vi "IL Turbo Speed.vi"(4 "Add to (Deny)":T1, 5 "Ignore (F)":bool, 6 "Range (>80%)":cluster{"Upper Limit":dbl, "Lower Limit":dbl}={"Upper Limit"=inf, "Lower Limit"=80.0}, 7 "Stop Self on IL? (T)":bool=TRUE, 8 "error in (no error)":errorcluster, 10 "IL Actions":refnum<class "IL Action.lvclass">[](array[class]), 11 "Interlock Chain in":refnum<class "Interlock Chain.lvclass">) -> (0 "error out":errorcluster, 2 "IL Turbo Valve":refnum<class "Interlock.lvclass">, 3 "Interlock Chain out":refnum<class "Interlock Chain.lvclass">)   [LabVIEW 2015, in "cRIO-Carbondioxide.lvlib" / "cRIO-CO2.lvlib" / "cRIO-CO2.lvclass"]
uses:
  cRIO-CO2.lvclass
  Interlocks/Interlock Chain/Interlock Chain.lvclass
  Interlocks/Controls/Add IL to -Enumerator.ctl
  Interlocks/Interlock/Interlock.lvclass
  Interlocks/IL Action/IL Action.lvclass
  Interlocks/Interlock DBL/Range/Interlock Range.lvclass
  Interlocks/Interlock DBL/Range/Interlock Range.lvclass/Interlock Range.ctl
  Interlocks/Interlock/Interlock.lvclass/Interlock.ctl
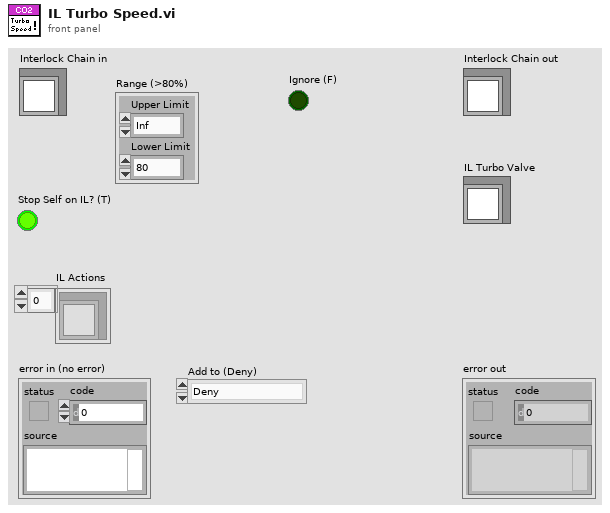
[diagram p1: front panel]
types:
  T1 = typedef "Add IL to -Enumerator.ctl" = enum16{"Deny", "Allow", "None"}
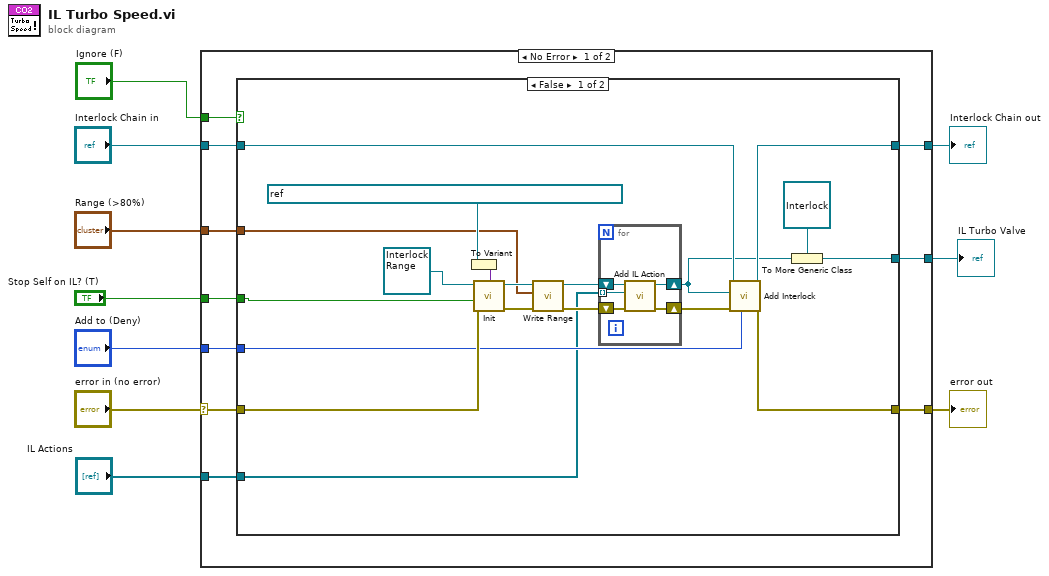
[diagram p0: block diagram]
diagram:
  n1 = case shown="No Error" "error in (no error)" {
    selector: "error in (no error)" -> [w18 w48]
    tunnel: [w17 w48] -> w9
    tunnel: [w19 w47] -> w7
    tunnel: "Interlock Chain in" -> [w20 w47]
    tunnel: "Range (>80%)" -> [w14 _]
    tunnel: "Add to (Deny)" -> [w16 _]
    tunnel: [w15 _] -> w4
    tunnel: "Stop Self on IL? (T)" -> [w13 _]
    tunnel: "Ignore (F)" -> [w12 _]
    tunnel: "IL Actions" -> [w11 _]
    frame No Error {
      n2 = case shown="False" w12 {
        tunnel: w20 -> [w35 w46]
        tunnel: [w34 w46] -> w19
        tunnel: w18 -> [w33 w45]
        tunnel: [w32 w45] -> w17
        tunnel: w16 -> [w31 _]
        tunnel: [w30 _] -> w15
        tunnel: w14 -> [w27 _]
        tunnel: w13 -> [w26 _]
        tunnel: w11 -> [w21 _]
        frame False {
          n3 = To Variant(anything=refnum<k21> "ni.var.psp://10.2.0.20/AMS Gas SHV/Vacuum/Turbo Speed" ("SHV")) -> (Variant=w28:variant)
          n4 = call-dynamic "Init.vi"("SHV"=w28, "error in (no error)"=w33, "Stop Self on IL? (T)"=w26, "Interlock in"=refnum<class "Interlock Range.lvclass"> refnum ("Interlock Range.lvclass")) -> ("error out"=w36:errorcluster, "Interlock out"=w37:refnum<class "Interlock Range.lvclass">)  [unwired: 6 in]
          n5 = call "Write Range.vi"("error in (no error)"=w36, "Range"=w27, "Interlock Bool in"=w37) -> ("error out"=w25:errorcluster, "Interlock Bool out"=w23:refnum<class "Interlock Range.lvclass">)  [unwired: 7 in]
          n6 = for {
            tunnel: w21 -> [w40] mode=indexing
            shift-right: [w43] -> w24
            shift-left: w25 -> [w44]
            shift-right: [w41] -> w22
            shift-left: w23 -> [w42]
            n7 = call "Add IL Action.vi"("error in (no error)"=w44, "IL Action in"=w40, "Interlock in"=w42) -> ("error out"=w43:errorcluster, "Interlock out"=w41:refnum<class "Interlock Range.lvclass">)  [unwired: 7 in]
          }
          n8 = call "Add Interlock.vi"("Add to (Deny)"=w31, "error in (no error)"=w24, "Interlock.lvclass"=w22, "Interlock Chain in"=w35) -> ("error out"=w32:errorcluster, "Interlock Chain out"=w34:refnum<class "Interlock Chain.lvclass">)  [unwired: 6 in]
          n9 = To More Generic Class(target class=refnum<class "Interlock.lvclass"> refnum ("Interlock.lvclass"), reference=w22) -> (generic class reference=w30:refnum<class "Interlock.lvclass">)
        }
        frame True {
        }
      }
    }
    frame Error {
    }
  }
  "error out" <- w9
  "Interlock Chain out" <- w7
  "IL Turbo Valve" <- w4
